vi "SELECT DATA.vi"(10 "DATA IN":string[][](array[string]), 11 "REFERENCES":T1) -> ()   [LabVIEW 2019]
uses:
  Controls/References Cluster.ctl
  Controls/Custom Calendar/Custom Calendar.xctl
  <vilib>/Utility/miscctls.llb/LVRowAndColumnTypeDef.ctl
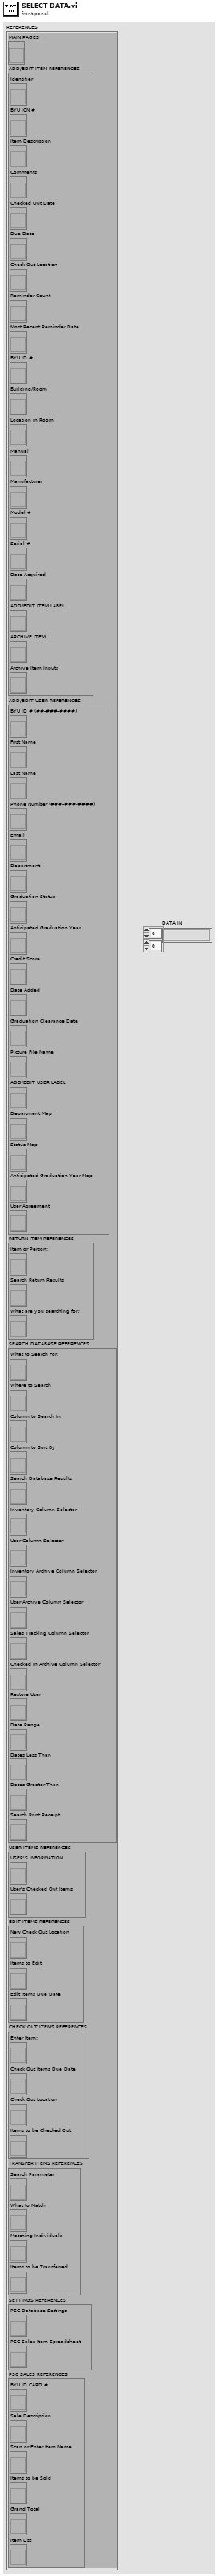
[diagram p1: front panel]
types:
  T1 = typedef "References Cluster.ctl" = cluster{"MAIN PAGES":refnum<vi>, "ADD/EDIT ITEM REFERENCES":cluster{"Identifier":refnum<vi>, "BYU ICN #":refnum<vi>, "Item Description":refnum<vi>, "Comments":refnum<vi>, "Checked Out Date":refnum<vi>, "Due Date":refnum<vi>, "Check Out Location":refnum<vi>, "Reminder Count":refnum<vi>, "Most Recent Reminder Date":refnum<vi>, "BYU ID #":refnum<vi>, "Building/Room":refnum<vi>, "Location in Room":refnum<vi>, "Manual":refnum<vi>, "Manufacturer":refnum<vi>, "Model #":refnum<vi>, "Serial #":refnum<vi>, "Date Acquired":refnum<vi>, "ADD/EDIT ITEM LABEL":refnum<vi>, "ARCHIVE ITEM":refnum<vi>, "Archive Item Inputs":refnum<vi>}, "ADD/EDIT USER REFERENCES":cluster{"BYU ID # (##-###-####)":refnum<vi>, "First Name":refnum<vi>, "Last Name":refnum<vi>, "Phone Number (###-###-####)":refnum<vi>, "Email":refnum<vi>, "Department":refnum<vi>, "Graduation Status":refnum<vi>, "Anticipated Graduation Year":refnum<vi>, "Credit Score":refnum<vi>, "Date Added":refnum<vi>, "Graduation Clearance Date":refnum<vi>, "Picture File Name":refnum<vi>, "ADD/EDIT USER LABEL":refnum<vi>, "Department Map":refnum<vi>, "Status Map":refnum<vi>, "Anticipated Graduation Year Map":refnum<vi>, "User Agreement":refnum<vi>}, "RETURN ITEM REFERENCES":cluster{"Item or Person:":refnum<vi>, "Search Return Results":refnum<vi>, "What are you searching for?":refnum<vi>}, "SEARCH DATABASE REFERENCES":cluster{"What to Search For:":refnum<vi>, "Where to Search":refnum<vi>, "Column to Search In":refnum<vi>, "Column to Sort By":refnum<vi>, "Search Database Results":refnum<vi>, "Inventory Column Selector":refnum<vi>, "User Column Selector":refnum<vi>, "Inventory Archive Column Selector":refnum<vi>, "User Archive Column Selector":refnum<vi>, "Sales Tracking Column Selector":refnum<vi>, "Checked In Archive Column Selector":refnum<vi>, "Restore User":refnum<vi>, "Date Range":refnum<vi>, "Dates Less Than":refnum<vi>, "Dates Greater Than":refnum<vi>, "Search Print Receipt":refnum<vi>}, "USER ITEMS REFERENCES":cluster{"USER'S INFORMATION":refnum<vi>, "User's Checked Out Items":refnum<vi>}, "EDIT ITEMS REFERENCES":cluster{"New Check Out Location":refnum<vi>, "Items to Edit":refnum<vi>, "Edit Items Due Date":refnum<vi>}, "CHECK OUT ITEMS REFERENCES":cluster{"Enter Item:":refnum<vi>, "Check Out Items Due Date":refnum<vi>, "Check Out Location":refnum<vi>, "Items to be Checked Out":refnum<vi>}, "TRANSFER ITEMS REFERENCES":cluster{"Search Parameter":refnum<vi>, "What to Match":refnum<vi>, "Matching Individuals":refnum<vi>, "Items to be Transferred":refnum<vi>}, "SETTINGS REFERENCES":cluster{"PSC Database Settings":refnum<vi>, "PSC Sales Item Spreadsheet":refnum<vi>}, "PSC SALES REFERENCES":cluster{"BYU ID CARD #":refnum<vi>, "Sale Description":refnum<vi>, "Scan or Enter Item Name":refnum<vi>, "Items to be Sold":refnum<vi>, "Grand Total":refnum<vi>, "Item List":refnum<vi>}}
  T2 = typedef "LVRowAndColumnTypeDef.ctl" = cluster{"Row":i32, "Column":i32}
  T3 = cluster{"What to Search For:":refnum<vi>, "Where to Search":refnum<vi>, "Column to Search In":refnum<vi>, "Column to Sort By":refnum<vi>, "Search Database Results":refnum<vi>, "Inventory Column Selector":refnum<vi>, "User Column Selector":refnum<vi>, "Inventory Archive Column Selector":refnum<vi>, "User Archive Column Selector":refnum<vi>, "Sales Tracking Column Selector":refnum<vi>, "Checked In Archive Column Selector":refnum<vi>, "Restore User":refnum<vi>, "Date Range":refnum<vi>, "Dates Less Than":refnum<vi>, "Dates Greater Than":refnum<vi>, "Search Print Receipt":refnum<vi>}
  T4 = cluster{"IDENTIFIER":bool, "BYU ICN #":bool, "ITEM":bool, "BUILDING/ROOM":bool, "LOCATION IN ROOM":bool, "MANUAL":bool, "MANUFACTURER":bool, "MODEL #":bool, "SERIAL #":bool, "DATE ACQUIRED":bool, "BYU ID":bool, "FIRST NAME":bool, "LAST NAME":bool, "CHECK OUT LOCATION":bool, "CHECKED OUT DATE":bool, "DUE DATE":bool, "REMINDER COUNT":bool, "MOST RECENT REMINDER DATE":bool, "COMMENTS":bool}
  T5 = cluster{"BYU ID #":bool, "FIRST NAME":bool, "LAST NAME":bool, "PHONE NUMBER":bool, "EMAIL":bool, "DEPARTMENT":bool, "GRADUATION STATUS":bool, "ANTICIPATED GRADUATION YEAR":bool, "CREDIT SCORE":bool, "DATE ADDED":bool, "GRADUATION CLEARANCE DATE":bool, "PICTURE FILE NAME":bool}
  T6 = cluster{"DATE DISPOSED":bool, "DISPOSAL METHOD":bool, "AUCTION #":bool, "DATE INVENTORY OFFICE EMAILED":bool, "DISPOSAL NOTES":bool, "IDENTIFIER":bool, "BYU ICN #":bool, "ITEM":bool, "COMMENTS":bool, "BUILDING/ROOM":bool, "LOCATION IN ROOM":bool, "MANUAL":bool, "MANUFACTURER":bool, "MODEL #":bool, "SERIAL #":bool, "DATE ACQUIRED":bool}
  T7 = cluster{"BYU ID #":bool, "FIRST NAME":bool, "LAST NAME":bool, "PHONE NUMBER":bool, "EMAIL":bool, "DEPARTMENT":bool, "STATUS":bool, "ANTICIPATED GRADUATION YEAR":bool, "CREDIT SCORE":bool, "DATE ADDED":bool, "GRADUATION CLEARANCE DATE":bool, "USER PROFILE PICTURE PATH":bool, "DATE ARCHIVED":bool}
  T8 = cluster{"ME #/ID #":bool, "BYU ICN #":bool, "ITEM DESCRIPTION":bool, "BUILDING/ROOM":bool, "LOCATION IN ROOM":bool, "MANUAL":bool, "MANUFACTURER":bool, "MODEL #":bool, "SERIAL #":bool, "DATE ACQUIRED":bool, "BYU ID #":bool, "FIRST NAME":bool, "LAST NAME":bool, "CHECK OUT LOCATION":bool, "CHECKED OUT DATE":bool, "DUE DATE":bool, "DATE RETURNED":bool, "REMINDER COUNT":bool, "MOST RECENT REMINDER DATE":bool, "COMMENTS":bool}
  T9 = cluster{"SALE ID #":bool, "BYU ID CARD #":bool, "Sale Description":bool, "Grand Total":bool, "SALE DATE":bool, "ITEM DESCRIPTION":bool, "ITEM UNIT PRICE":bool, "ITEM TOTAL PRICE":bool, "ITEM QUANTITY":bool, "SALE SEMESTER":bool}
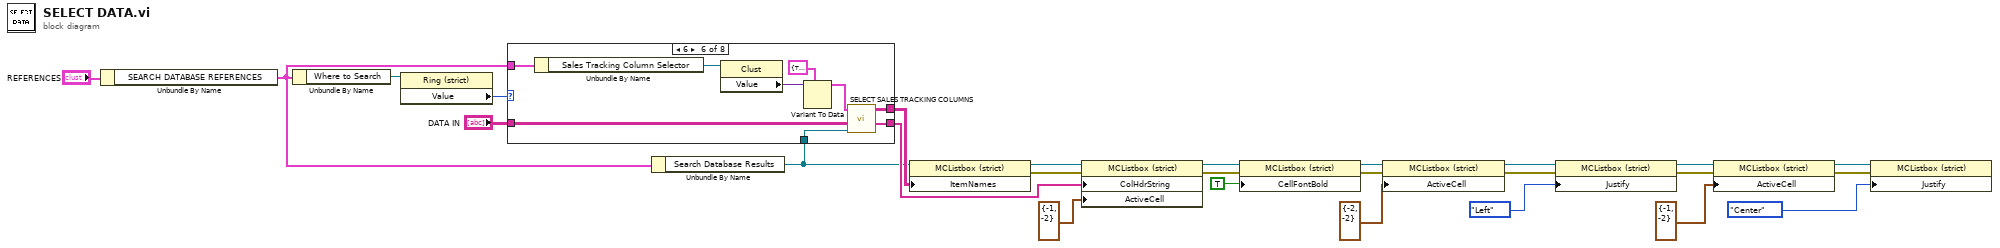
[diagram p0: block diagram]
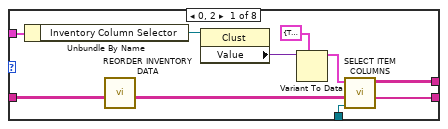
[diagram p2: hidden frame]
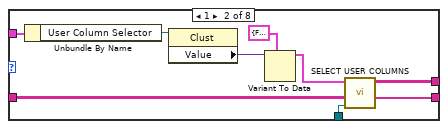
[diagram p3: hidden frame]
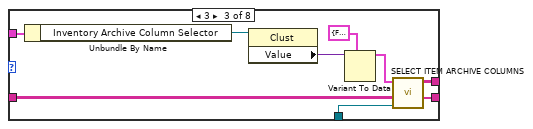
[diagram p4: hidden frame]
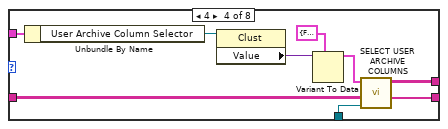
[diagram p5: hidden frame]
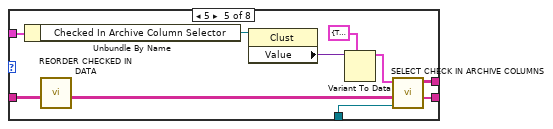
[diagram p6: hidden frame]
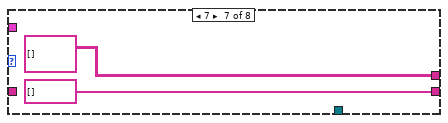
[diagram p7: hidden frame]
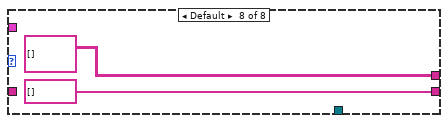
[diagram p8: hidden frame]
diagram:
  n1 = Unbundle By Name("REFERENCES") -> ("SEARCH DATABASE REFERENCES"=w21:T3)
  n2 = Unbundle By Name(w21) -> ("Where to Search"=w26:refnum<vi>)
  n3 = property class="Ring (strict)"(reference=w26) -> ("Value"=w25:u16)  [unwired: 1 in, 2 out]
  n4 = Unbundle By Name(w21) -> ("Search Database Results"=w1:refnum<vi>)
  n5 = case shown="6" w25 {
    tunnel: w21 -> [w36 w43 w53 w59 w72 w82 _ _]
    tunnel: [w32 w41 w50 w61 w70 w78 string[][] [] ("DATA OUT") string[][] [] ("DATA OUT")] -> w24
    tunnel: [w31 w40 w49 w58 w69 w77 string[] [] ("DATA OUT") string[] [] ("DATA OUT")] -> w2
    tunnel: "DATA IN" -> [w29 w39 w48 w57 w65 w76 _ _]
    tunnel: w1 -> [w30 w38 w46 w55 w68 w75 _ _]
    frame 0, 2 {
      n6 = Unbundle By Name(w36) -> ("Inventory Column Selector"=w35:refnum<vi>)
      n7 = call "REORDER INVENTORY DATA.vi"("DATA IN"=w29) -> ("DATA OUT"=w28:string[][])  [unwired: 10 in]
      n8 = property class="Clust"(reference=w35) -> ("Value"=w34:variant)  [unwired: 1 in, 2 out]
      n9 = Variant To Data(type=T4 {"IDENTIFIER"=TRUE, "BYU ICN #"=TRUE, "ITEM"=TRUE, "BUILDING/ROOM"=FALSE, "LOCATION IN ROOM"=FALSE, "MANUAL"=TRUE, "MANUFACTURER"=FALSE, "MODEL #"=FALSE, "SERIAL #"=FALSE, "DATE ACQUIRED"=FALSE, "BYU ID"=TRUE, "FIRST NAME"=TRUE, "LAST NAME"=TRUE, "CHECK OUT LOCATION"=TRUE, "CHECKED OUT DATE"=TRUE, "DUE DATE"=TRUE, "REMINDER COUNT"=TRUE, "MOST RECENT REMINDER DATE"=TRUE, "COMMENTS"=FALSE} ("Inventory Column Selector"), Variant=w34) -> (data=w33:T4)  [unwired: 1 in, 1 out]
      n10 = call "SELECT ITEM COLUMNS.vi"("Inventory Column Selector"=w33, "DATA IN"=w28, "Search Database Results"=w30) -> ("DATA OUT"=w32:string[][], "HEADERS OUT"=w31:string[])  [unwired: 6 in]
    }
    frame 1 {
      n11 = Unbundle By Name(w43) -> ("User Column Selector"=w45:refnum<vi>)
      n12 = property class="Clust"(reference=w45) -> ("Value"=w44:variant)  [unwired: 1 in, 2 out]
      n13 = Variant To Data(type=T5 {"BYU ID #"=FALSE, "FIRST NAME"=FALSE, "LAST NAME"=FALSE, "PHONE NUMBER"=FALSE, "EMAIL"=FALSE, "DEPARTMENT"=FALSE, "GRADUATION STATUS"=FALSE, "ANTICIPATED GRADUATION YEAR"=FALSE, "CREDIT SCORE"=FALSE, "DATE ADDED"=FALSE, "GRADUATION CLEARANCE DATE"=FALSE, "PICTURE FILE NAME"=FALSE} ("User Column Selector"), Variant=w44) -> (data=w42:T5)  [unwired: 1 in, 1 out]
      n14 = call "SELECT USER COLUMNS.vi"("Search Database Results"=w38, "DATA IN"=w39, "User Column Selector"=w42) -> ("HEADERS OUT"=w40:string[], "DATA OUT"=w41:string[][])  [unwired: 7 in]
    }
    frame 3 {
      n15 = Unbundle By Name(w53) -> ("Inventory Archive Column Selector"=w52:refnum<vi>)
      n16 = property class="Clust"(reference=w52) -> ("Value"=w54:variant)  [unwired: 1 in, 2 out]
      n17 = Variant To Data(type=T6 {"DATE DISPOSED"=FALSE, "DISPOSAL METHOD"=FALSE, "AUCTION #"=FALSE, "DATE INVENTORY OFFICE EMAILED"=FALSE, "DISPOSAL NOTES"=FALSE, "IDENTIFIER"=FALSE, "BYU ICN #"=FALSE, "ITEM"=FALSE, "COMMENTS"=FALSE, "BUILDING/ROOM"=FALSE, "LOCATION IN ROOM"=FALSE, "MANUAL"=FALSE, "MANUFACTURER"=FALSE, "MODEL #"=FALSE, "SERIAL #"=FALSE, "DATE ACQUIRED"=FALSE} ("Inventory Archive Column Selector"), Variant=w54) -> (data=w51:T6)  [unwired: 1 in, 1 out]
      n18 = call "SELECT ITEM ARCHIVE COLUMNS.vi"("Search Database Results"=w46, "DATA IN"=w48, "Inventory Archive Column Selector"=w51) -> ("HEADERS OUT"=w49:string[], "DATA OUT"=w50:string[][])  [unwired: 7 in]
    }
    frame 4 {
      n19 = Unbundle By Name(w59) -> ("User Archive Column Selector"=w62:refnum<vi>)
      n20 = property class="Clust"(reference=w62) -> ("Value"=w63:variant)  [unwired: 1 in, 2 out]
      n21 = Variant To Data(type=T7 {"BYU ID #"=FALSE, "FIRST NAME"=FALSE, "LAST NAME"=FALSE, "PHONE NUMBER"=FALSE, "EMAIL"=FALSE, "DEPARTMENT"=FALSE, "STATUS"=FALSE, "ANTICIPATED GRADUATION YEAR"=FALSE, "CREDIT SCORE"=FALSE, "DATE ADDED"=FALSE, "GRADUATION CLEARANCE DATE"=FALSE, "USER PROFILE PICTURE PATH"=FALSE, "DATE ARCHIVED"=FALSE} ("User Archive Column Selector"), Variant=w63) -> (data=w60:T7)  [unwired: 1 in, 1 out]
      n22 = call "SELECT USER ARCHIVE COLUMNS.vi"("Search Database Results"=w55, "DATA IN"=w57, "User Archive Column Selector"=w60) -> ("HEADERS OUT"=w58:string[], "DATA OUT"=w61:string[][])  [unwired: 7 in]
    }
    frame 5 {
      n23 = Unbundle By Name(w72) -> ("Checked In Archive Column Selector"=w71:refnum<vi>)
      n24 = call "REORDER CHECKED IN DATA.vi"("DATA IN"=w65) -> ("DATA OUT"=w64:string[][])  [unwired: 10 in]
      n25 = property class="Clust"(reference=w71) -> ("Value"=w73:variant)  [unwired: 1 in, 2 out]
      n26 = Variant To Data(type=T8 {"ME #/ID #"=TRUE, "BYU ICN #"=TRUE, "ITEM DESCRIPTION"=TRUE, "BUILDING/ROOM"=FALSE, "LOCATION IN ROOM"=FALSE, "MANUAL"=TRUE, "MANUFACTURER"=FALSE, "MODEL #"=FALSE, "SERIAL #"=FALSE, "DATE ACQUIRED"=FALSE, "BYU ID #"=TRUE, "FIRST NAME"=TRUE, "LAST NAME"=TRUE, "CHECK OUT LOCATION"=TRUE, "CHECKED OUT DATE"=TRUE, "DUE DATE"=TRUE, "DATE RETURNED"=TRUE, "REMINDER COUNT"=FALSE, "MOST RECENT REMINDER DATE"=FALSE, "COMMENTS"=FALSE} ("Checked In Archive Selector"), Variant=w73) -> (data=w66:T8)  [unwired: 1 in, 1 out]
      n27 = call "SELECT CHECK IN ARCHIVE COLUMNS.vi"("Search Database Results"=w68, "DATA IN"=w64, "Checked In Archive Selector"=w66) -> ("HEADERS OUT"=w69:string[], "DATA OUT"=w70:string[][])  [unwired: 7 in]
    }
    frame 6 {
      n28 = Unbundle By Name(w82) -> ("Sales Tracking Column Selector"=w81:refnum<vi>)
      n29 = property class="Clust"(reference=w81) -> ("Value"=w80:variant)  [unwired: 1 in, 2 out]
      n30 = Variant To Data(type=T9 {"SALE ID #"=TRUE, "BYU ID CARD #"=TRUE, "Sale Description"=TRUE, "Grand Total"=TRUE, "SALE DATE"=TRUE, "ITEM DESCRIPTION"=TRUE, "ITEM UNIT PRICE"=TRUE, "ITEM TOTAL PRICE"=TRUE, "ITEM QUANTITY"=TRUE, "SALE SEMESTER"=TRUE} ("Sales Tracking Column Selector"), Variant=w80) -> (data=w79:T9)  [unwired: 1 in, 1 out]
      n31 = call "SELECT SALES TRACKING COLUMNS.vi"("Search Database Results"=w75, "DATA IN"=w76, "Sales Tracking Column Selector"=w79) -> ("HEADERS OUT"=w77:string[], "DATA OUT"=w78:string[][])  [unwired: 7 in]
    }
    frame 7 {
    }
    frame Default {
    }
  }
  n32 = property class="MCListbox (strict)"(reference=w1, "ItemNames"=w24) -> (reference out=w4:refnum<vi>, error out=w3:errorcluster)  [unwired: 1 in]
  n33 = property class="MCListbox (strict)"(reference=w4, error in=w3, "ColHdrString"=w2, "ActiveCell"=T2 {"Row"=-1, "Column"=-2} ("Active Cell:Active Cell")) -> (reference out=w19:refnum<vi>, error out=w18:errorcluster)
  n34 = property class="MCListbox (strict)"(reference=w19, error in=w18, "CellFontBold"=TRUE ("Active Cell:Cell Font:Bold")) -> (reference out=w16:refnum<vi>, error out=w15:errorcluster)
  n35 = property class="MCListbox (strict)"(reference=w16, error in=w15, "ActiveCell"=T2 {"Row"=-2, "Column"=-2} ("Active Cell:Active Cell")) -> (reference out=w13:refnum<vi>, error out=w12:errorcluster)
  n36 = property class="MCListbox (strict)"(reference=w13, error in=w12, "Justify"=enum16{"Left", "Center", "Right"}."Left" ("Active Cell:Cell Justification")) -> (reference out=w8:refnum<vi>, error out=w7:errorcluster)
  n37 = property class="MCListbox (strict)"(reference=w8, error in=w7, "ActiveCell"=T2 {"Row"=-1, "Column"=-2} ("Active Cell:Active Cell")) -> (reference out=w9:refnum<vi>, error out=w10:errorcluster)
  n38 = property class="MCListbox (strict)"(reference=w9, error in=w10, "Justify"=enum16{"Left", "Center", "Right"}."Center" ("Active Cell:Cell Justification")) -> ()  [unwired: 2 out]
